vi "SimpleWhile.vi"(10 "process variable":dbl format="%.2f", 11 "setpoint":dbl format="%.2f") -> (2 "output":dbl format="%.2f")   [LabVIEW 2012]
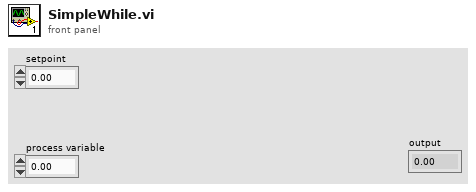
[diagram p1: front panel]
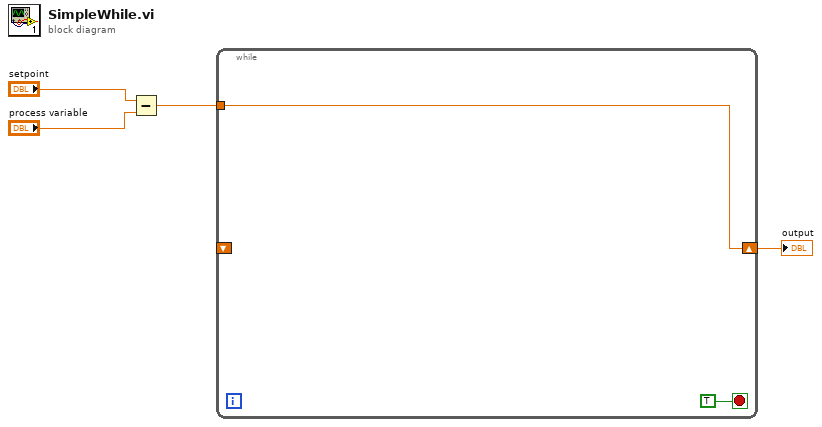
[diagram p0: block diagram]
diagram:
  n1 = Subtract(x="setpoint", y="process variable") -> (x-y=w2:dbl)
  n2 = while {
    shift-right: [w5] -> w1
    shift-left: _ -> [_]
    tunnel: w2 -> [w5]
    stop <- TRUE stop-if-true
  }
  "output" <- w1
